vi "Edit.vi"() -> ()   [LabVIEW 2021]
panel:
  out "Discount":dbl
  out "Bill":dbl
  out "Discount percentage":string
  out "Rs.":dbl
  out "Rs.":dbl
  out "Rs.":dbl
  out "Rs.":dbl
  out "Rs.":dbl
  in  "Carrot":bool
  in  "kg":dbl
  in  "Cabege":bool
  in  "kg":dbl
  in  "Bringle":bool
  in  "kg":dbl
  in  "Beans":bool
  in  "kg":dbl
  in  "Leeks":bool
  in  "kg":dbl
  out "Total Bill":dbl
  in  "Banana":bool
  out "Rs.":dbl
  in  "Apple":bool
  out "Rs.":dbl
  in  "kg":dbl
  in  "Orange":bool
  out "Rs.":dbl
  in  "kg":dbl
  in  "Graps":bool
  out "Rs.":dbl
  in  "kg":dbl
  in  "Papaya":bool
  in  "kg":dbl
  out "Rs.":dbl
  in  "kg":dbl
  # "Price per 1kg (Rs.)"
  # "Quantities(kg)"
  # "Vegetables"
  # "Fruits"
  # "Bill details"
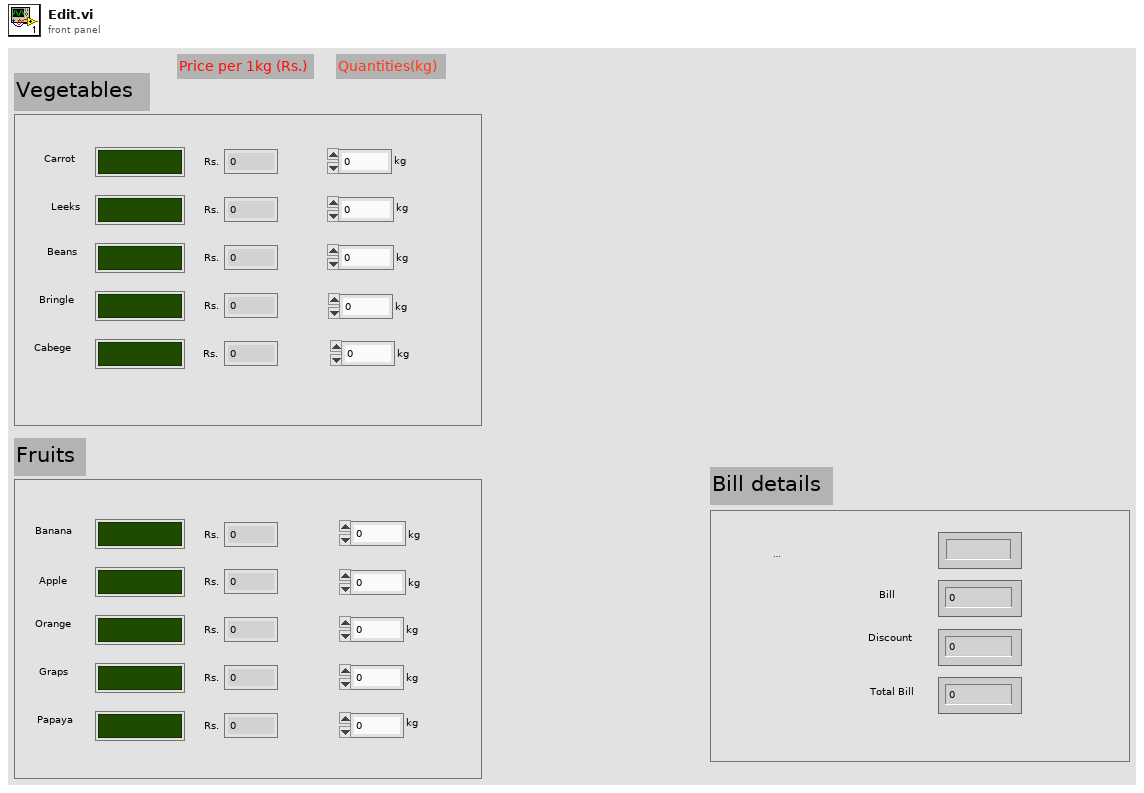
[diagram p1: front panel]
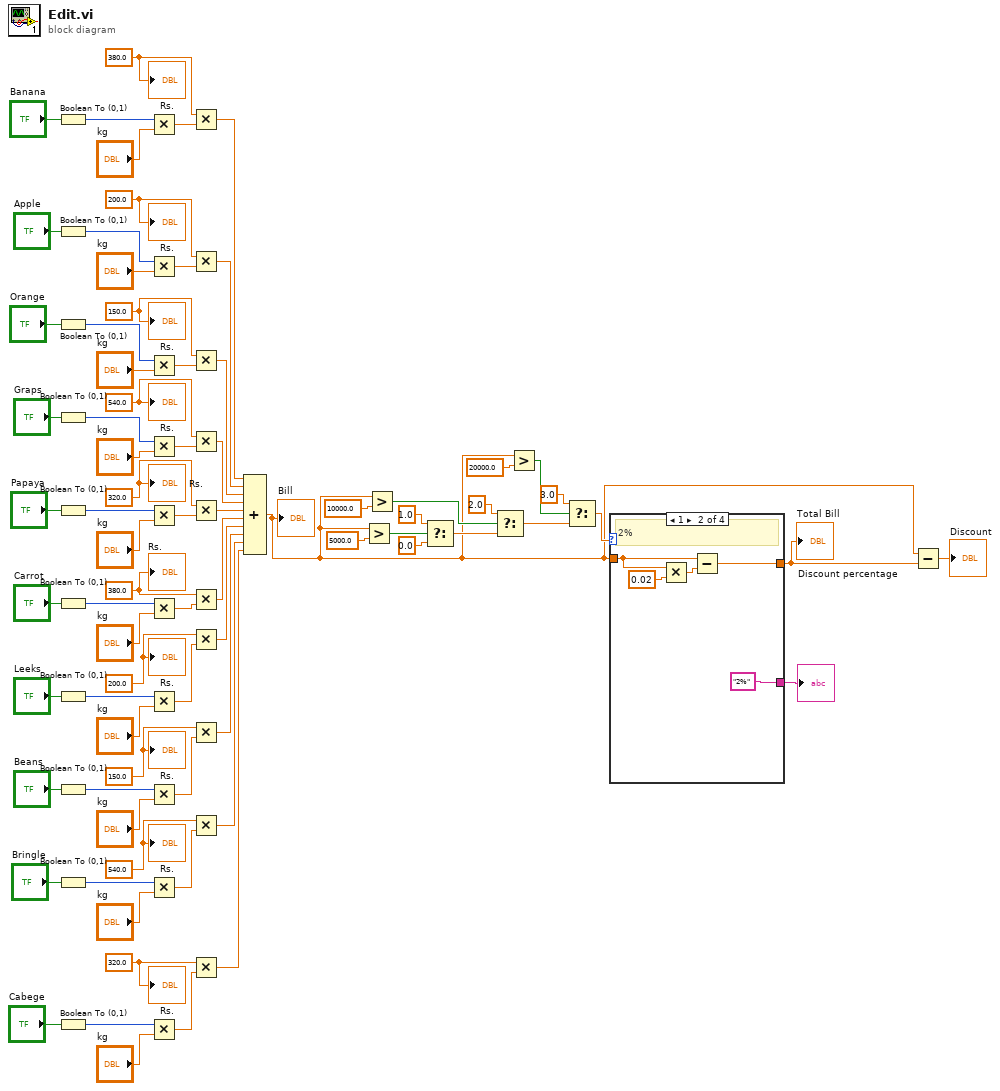
[diagram p0: block diagram]
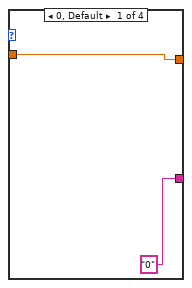
[diagram p2: hidden frame]
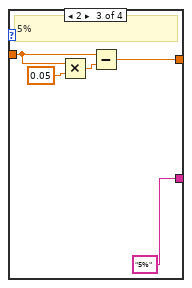
[diagram p3: hidden frame]
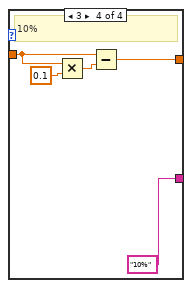
[diagram p4: hidden frame]
diagram:
  w54 = 320.0 ("price")
  w61 = 540.0 ("price")
  w64 = 150.0 ("price")
  w71 = 200.0 ("price")
  w74 = 380.0 ("price")
  w29 = 320.0 ("price")
  w36 = 540.0 ("price")
  w39 = 150.0 ("price")
  w46 = 200.0 ("price")
  w49 = 380.0 ("price")
  n1 = Boolean To (0,1)(Boolean="Banana") -> (0, 1=w76:i16)
  n2 = Boolean To (0,1)(Boolean="Apple") -> (0, 1=w69:i16)
  n3 = Boolean To (0,1)(Boolean="Orange") -> (0, 1=w66:i16)
  n4 = Boolean To (0,1)(Boolean="Graps") -> (0, 1=w59:i16)
  n5 = Boolean To (0,1)(Boolean="Papaya") -> (0, 1=w56:i16)
  n6 = Boolean To (0,1)(Boolean="Carrot") -> (0, 1=w51:i16)
  n7 = Boolean To (0,1)(Boolean="Leeks") -> (0, 1=w44:i16)
  n8 = Boolean To (0,1)(Boolean="Beans") -> (0, 1=w41:i16)
  n9 = Boolean To (0,1)(Boolean="Bringle") -> (0, 1=w34:i16)
  n10 = Boolean To (0,1)(Boolean="Cabege") -> (0, 1=w31:i16)
  n11 = Multiply(x=w76, y="kg") -> (x*y=w73:dbl)
  n12 = Multiply(x=w69, y="kg") -> (x*y=w72:dbl)
  n13 = Multiply(x=w66, y="kg") -> (x*y=w63:dbl)
  n14 = Multiply(x=w59, y="kg") -> (x*y=w62:dbl)
  n15 = Multiply(x=w56, y="kg") -> (x*y=w53:dbl)
  n16 = Multiply(x=w51, y="kg") -> (x*y=w48:dbl)
  n17 = Multiply(x=w44, y="kg") -> (x*y=w47:dbl)
  n18 = Multiply(x=w41, y="kg") -> (x*y=w38:dbl)
  n19 = Multiply(x=w34, y="kg") -> (x*y=w37:dbl)
  n20 = Multiply(x=w31, y="kg") -> (x*y=w28:dbl)
  n21 = Multiply(x=w74, y=w73) -> (x*y=w11:dbl)
  n22 = Multiply(x=w71, y=w72) -> (x*y=w10:dbl)
  n23 = Multiply(x=w64, y=w63) -> (x*y=w9:dbl)
  n24 = Multiply(x=w61, y=w62) -> (x*y=w8:dbl)
  n25 = Multiply(x=w54, y=w53) -> (x*y=w7:dbl)
  n26 = Multiply(x=w49, y=w48) -> (x*y=w6:dbl)
  n27 = Multiply(x=w46, y=w47) -> (x*y=w5:dbl)
  n28 = Multiply(x=w39, y=w38) -> (x*y=w4:dbl)
  n29 = Multiply(x=w36, y=w37) -> (x*y=w3:dbl)
  n30 = Multiply(x=w29, y=w28) -> (x*y=w2:dbl)
  n31 = Compound Arithmetic op=ADD(w11, w10, w9, w8, w7, w6, w5, w4, w3, w2) -> (w1:dbl)
  "Bill" <- w1
  n32 = Greater?(x=w1, y=5000.0) -> (0:w16:bool)
  n33 = Greater?(x=w1, y=10000.0) -> (0:w15:bool)
  n34 = Select(t=1.0, s=w16, f=0.0) -> (s? t:f=w20:dbl)
  n35 = Select(t=2.0, s=w15, f=w20) -> (s? t:f=w19:dbl)
  n36 = Greater?(x=w1, y=20000.0) -> (0:w14:bool)
  n37 = Select(t=3.0, s=w14, f=w19) -> (s? t:f=w18:dbl)
  n38 = case shown="1" w18 {
    tunnel: [w79 w83 w86 w91] -> w13
    tunnel: w1 -> [w79 w82 w87 w92]
    tunnel: ["0" ("discount") "2%" ("discount") "5%" ("discount") "10%" ("discount")] -> w17
    frame 0, Default {
    }
    frame 1 {
      # "2%"
      n39 = Multiply(x=w82, y=0.02) -> (x*y=w80:dbl)
      n40 = Subtract(x=w82, y=w80) -> (x-y=w83:dbl)
    }
    frame 2 {
      # "5%"
      n41 = Multiply(x=w87, y=0.05) -> (x*y=w88:dbl)
      n42 = Subtract(x=w87, y=w88) -> (x-y=w86:dbl)
    }
    frame 3 {
      # "10%"
      n43 = Multiply(x=w92, y=0.1) -> (x*y=w93:dbl)
      n44 = Subtract(x=w92, y=w93) -> (x-y=w91:dbl)
    }
  }
  "Total Bill" <- w13
  "Discount percentage" <- w17
  n45 = Subtract(x=w1, y=w13) -> (x-y=→"Discount":dbl)
  "Rs." <- w49
  "Rs." <- w46
  "Rs." <- w39
  "Rs." <- w36
  "Rs." <- w29
  "Rs." <- w74
  "Rs." <- w71
  "Rs." <- w64
  "Rs." <- w61
  "Rs." <- w54
